vi "Untitled 1.vi"() -> ()   [LabVIEW 2020]
panel:
  in  "Boolean":bool
  in  "working directory 2":path=path ""
  in  "working directory":path=path ""
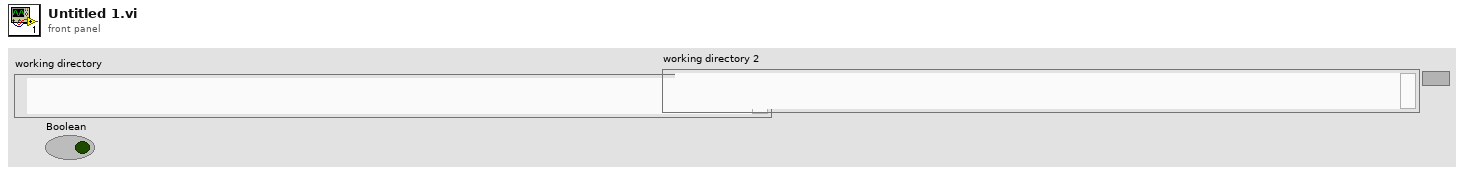
[diagram p1: front panel]
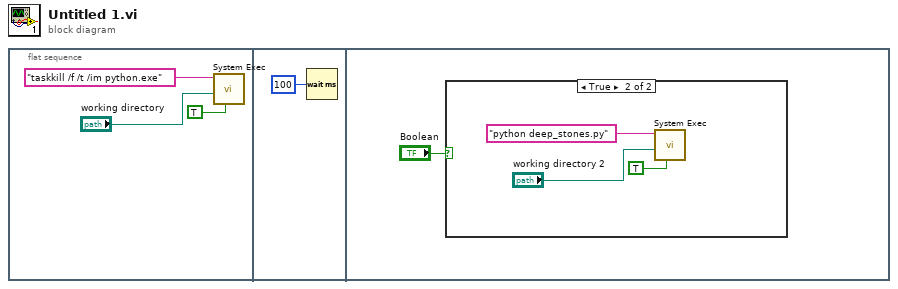
[diagram p0: block diagram]
diagram:
  n1 = flat-sequence {
    frame #0 {
      n2 = call <vilib>:"System Exec.vi"("run minimized? (F)"=TRUE, "working directory"="working directory", "command line"="taskkill /f /t /im python.exe") -> ()  [unwired: 5 in, 4 out]
    }
    frame #1 {
      n3 = Wait (ms)(milliseconds to wait=u32 100) -> ()  [unwired: 1 out]
    }
    frame #2 {
      n4 = case shown="True" "Boolean" {
        frame False {
        }
        frame True {
          n5 = call <vilib>:"System Exec.vi"("run minimized? (F)"=TRUE, "working directory"="working directory 2", "command line"="python deep_stones.py") -> ()  [unwired: 5 in, 4 out]
        }
      }
    }
  }
